vi "Utility_CalculatePointsXY.vi"(0 "trajectory":T2, 1 "reset":bool, 5 "Posture(n-1)":T1, 7 "linearV":dbl, 12 "dt":dbl) -> (4 "index":i32, 6 "fractional index":dbl, 8 "desired LinearV":dbl, 15 "cross 2 elements":bool)   [LabVIEW 2017]
uses:
  Trajectory.ctl
  VehiclePosture.ctl
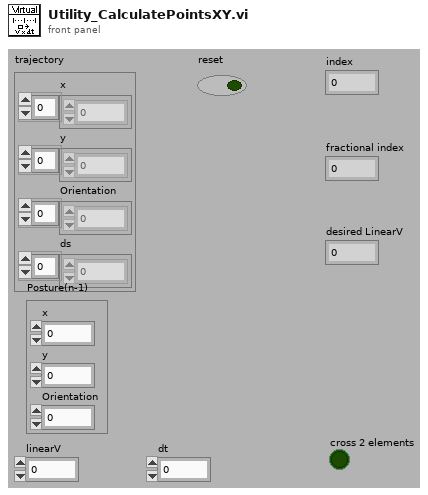
[diagram p1: front panel]
types:
  T1 = typedef "VehiclePosture.ctl" = cluster{"x":dbl, "y":dbl, "Orientation":dbl}
  T2 = typedef "Trajectory.ctl" = cluster{"x":dbl[], "y":dbl[], "Orientation":dbl[], "ds":dbl[]}
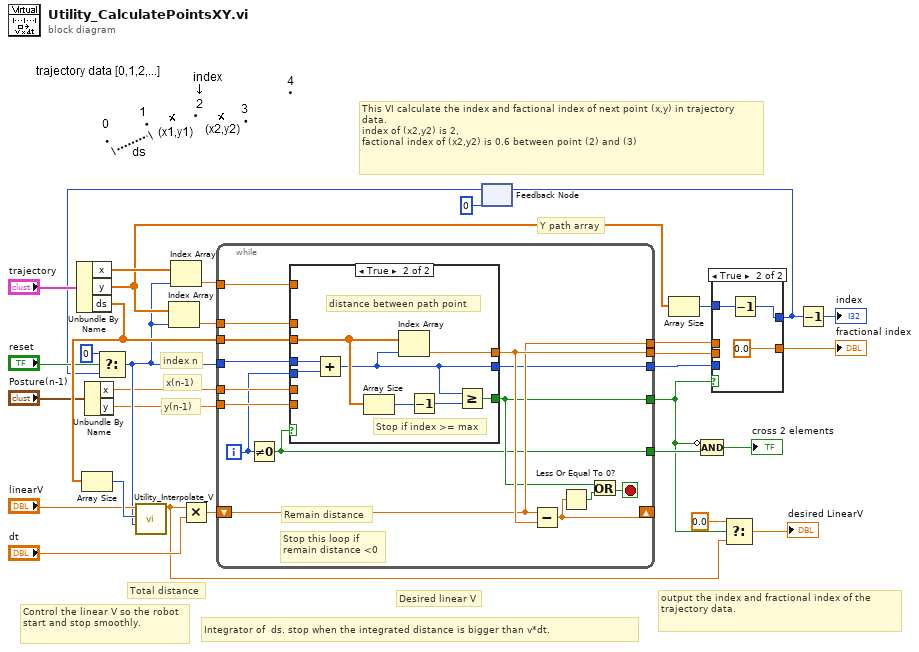
[diagram p0: block diagram]
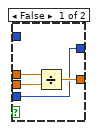
[diagram p2: hidden frame]
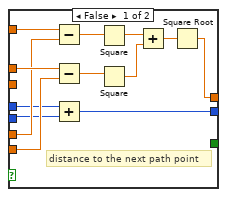
[diagram p3: hidden frame]
diagram:
  # "output the index and fractional index of the trajectory data."
  # "Integrator of  ds. stop when the integrated distance is bigger than v*dt."
  # "Control the linear V so the robot start and stop smoothly."
  # "This VI calculate the index and factional index of next point (x,y) in trajectory data.\nindex of (x2,y2) is 2,\nfactional index of (x2,y2) is 0.6 between point (2) and (3)"
  # "Y path array"
  # "Desired linear V"
  # "Total distance"
  # "index n"
  # "y(n-1)"
  # "x(n-1)"
  n1 = Unbundle By Name("trajectory") -> ("x"=w28:dbl[], "y"=w23:dbl[], "ds"=w19:dbl[])
  n2 = Array Size(array=w19) -> (size(s)=w18:i32)
  n3 = Unbundle By Name("Posture(n-1)") -> ("x"=w6:dbl, "y"=w5:dbl)
  n4 = feedback #1(0) -> (w10:i32)
  n5 = Select(t=0, s="reset", f=w10) -> (s? t:f=w8:i32)
  n6 = call "Utility_Interpolate_V.vi"("index"=w8, "length"=w18, "linear velocity"="linearV") -> ("linear velocity"=w2:dbl)  [unwired: 8 in]
  n7 = Index Array(array=w23, index=w8) -> (element=w27:dbl)
  n8 = Index Array(array=w28, index=w8) -> (element=w26:dbl)
  n9 = Multiply(x=w2, y="dt") -> (x*y=w31:dbl)
  n10 = while {
    tunnel: w19 -> [w46]
    tunnel: w8 -> [w45]
    tunnel: w26 -> [w44]
    tunnel: w27 -> [w43]
    tunnel: w6 -> [w42]
    tunnel: w5 -> [w41]
    shift-right: [w40] -> _
    shift-left: w31 -> [w38]
    tunnel: [w39] -> w25
    tunnel: [w38] -> w30
    tunnel: [w37] -> w24
    tunnel: [w34] -> w4
    tunnel: [w32] -> w20
    i -> [w33]
    stop <- w35 stop-if-true
    # "Stop this loop if \nremain distance <0"
    # "Remain distance"
    n11 = Not Equal To 0?(x=w33) -> (x != 0?=w32:bool)
    n12 = case shown="True" w32 {
      tunnel: w46 -> [_ w64]
      tunnel: w45 -> [w49 w67]
      tunnel: w33 -> [w48 w66]
      tunnel: w44 -> [w54 _]
      tunnel: w43 -> [w53 _]
      tunnel: w42 -> [w52 _]
      tunnel: w41 -> [w51 _]
      tunnel: [w50 w65] -> w39
      tunnel: [w47 w63] -> w37
      tunnel: [_ w62] -> w34
      frame False {
        # "distance to the next path point"
        n13 = Subtract(x=w54, y=w52) -> (x-y=w55:dbl)
        n14 = Subtract(x=w53, y=w51) -> (x-y=w56:dbl)
        n15 = Add(x=w49, y=w48) -> (x+y=w47:i32)
        n16 = Square(x=w55) -> (x^2=w57:dbl)
        n17 = Square(x=w56) -> (x^2=w58:dbl)
        n18 = Add(x=w57, y=w58) -> (x+y=w59:dbl)
        n19 = Square Root(x=w59) -> (sqrt(x)=w50:dbl)
      }
      frame True {
        # "Stop if index >= max"
        # "distance between path point"
        n20 = Add(x=w67, y=w66) -> (x+y=w63:i32)
        n21 = Array Size(array=w64) -> (size(s)=w61:i32)
        n22 = Index Array(array=w64, index=w63) -> (element=w65:dbl)
        n23 = Decrement(x=w61) -> (x-1=w60:i32)
        n24 = Greater Or Equal?(x=w63, y=w60) -> (x >= y?=w62:bool)
      }
    }
    n25 = Subtract(x=w38, y=w39) -> (x-y=w40:dbl)
    n26 = Less Or Equal To 0?(x=w40) -> (x <= 0?=w36:bool)
    n27 = Or(x=w34, y=w36) -> (x .or. y?=w35:bool)
  }
  n28 = Array Size(array=w23) -> (size(s)=w22:i32)
  n29 = Compound Arithmetic op=AND(invert w4, w20) -> (→"cross 2 elements":bool)
  n30 = case shown="True" w4 {
    tunnel: w30 -> [w71 _]
    tunnel: [w70 0.0] -> w13
    tunnel: w25 -> [w69 _]
    tunnel: w24 -> [w68 _]
    tunnel: [w68 w72] -> w21
    tunnel: w22 -> [_ w73]
    frame False {
      n31 = Divide(x=w71, y=w69) -> (x/y=w70:dbl)
    }
    frame True {
      n32 = Decrement(x=w73) -> (x-1=w72:i32)
    }
  }
  "fractional index" <- w13
  n33 = feedback-in #1(w21) -> ()
  n34 = Select(t=0.0, s=w4, f=w2) -> (s? t:f=→"desired LinearV":dbl)
  n35 = Decrement(x=w21) -> (x-1=→"index":i32)
